vi "FILE READ FROM CSV.vi"(0 "File Path":string="C:\\data\\07_34_08_PM_01_July_2026\\07_34_08_PM_01_July_202607_34_08_PM_01_July_2026.csv", 5 "X-AXIS":u16(ring) items=["None", "Time ( Sec )", "Normal Load ( N )", "Frictional Force ( N )", "Coefficient of Friction", "Depth ( Microns )", "Speed ( RPM )", "Frequency ( Hz )", "Angle ( Degree )", "Cyclic Friction Force ( N )", "Cyclic Co efficient Friction ", "Stage temperature ( Degree celcius )", "Sample temperature ( Degree celcius )", "Stroke Length ( mm )", "Scratch Speed ( mm/sec )", "Amb Humidity ( % Rh ) ", "Amb Temperature (Deg C)", "Acoustic (mV)", "Mx (Nm)", "My (Nm)", "Mz (Nm)", "Humidity ( % Rh )", "Sliding Distance (mm)", "Wear Track Diameter (mm)", "Fx(N)", "Fy(N)", "MTM BallSpeed (RPM)", "MTM DiscSpeed (RPM)", "Entrainment Speed", "Slide Role", "Slip(%)", "Rotary Speed (m/sec)", "MTM Ball Speed (m/sec)", "MTM Disc Speed (m/sec)", "ECR (ohms)"], 9 "Y-AXIS":u16(ring) items=["None", "Time ( Sec )", "Normal Load ( N )", "Frictional Force ( N )", "Coefficient of Friction", "Depth ( Microns )", "Speed ( RPM )", "Frequency ( Hz )", "Angle ( Degree )", "Cyclic Friction Force ( N )", "Cyclic Co efficient Friction ", "Stage temperature ( Degree celcius )", "Sample temperature ( Degree celcius )", "Stroke Length ( mm )", "Scratch Speed ( mm/sec )", "Amb Humidity ( % Rh ) ", "Amb Temperature (Deg C)", "Acoustic (mV)", "Mx (Nm)", "My (Nm)", "Mz (Nm)", "Humidity ( % Rh )", "Sliding Distance (mm)", "Wear Track Diameter (mm)", "Fx(N)", "Fy(N)", "MTM BallSpeed (RPM)", "MTM DiscSpeed (RPM)", "Entrainment Speed", "Slide Role", "Slip(%)", "Rotary Speed (m/sec)", "MTM Ball Speed (m/sec)", "MTM Disc Speed (m/sec)", "ECR (ohms)"], 11 "error in (no error)":errorcluster) -> (4 "output cluster":cluster{"X":dbl[], "Y":dbl[]}, 6 "mean":dbl format="%0.2f", 8 "standard deviation":dbl format="%0.2f", 10 "variance":dbl format="%0.2f", 15 "error out":errorcluster)   [LabVIEW 2025]
uses:
  <vilib>/Analysis/NI_AALBase.lvlib
panel:
  # "C:\\data\\07_34_08_PM_01_July_2026\\07_34_08_PM_01_July_202607_34_08_PM_01_July_2026.csv"
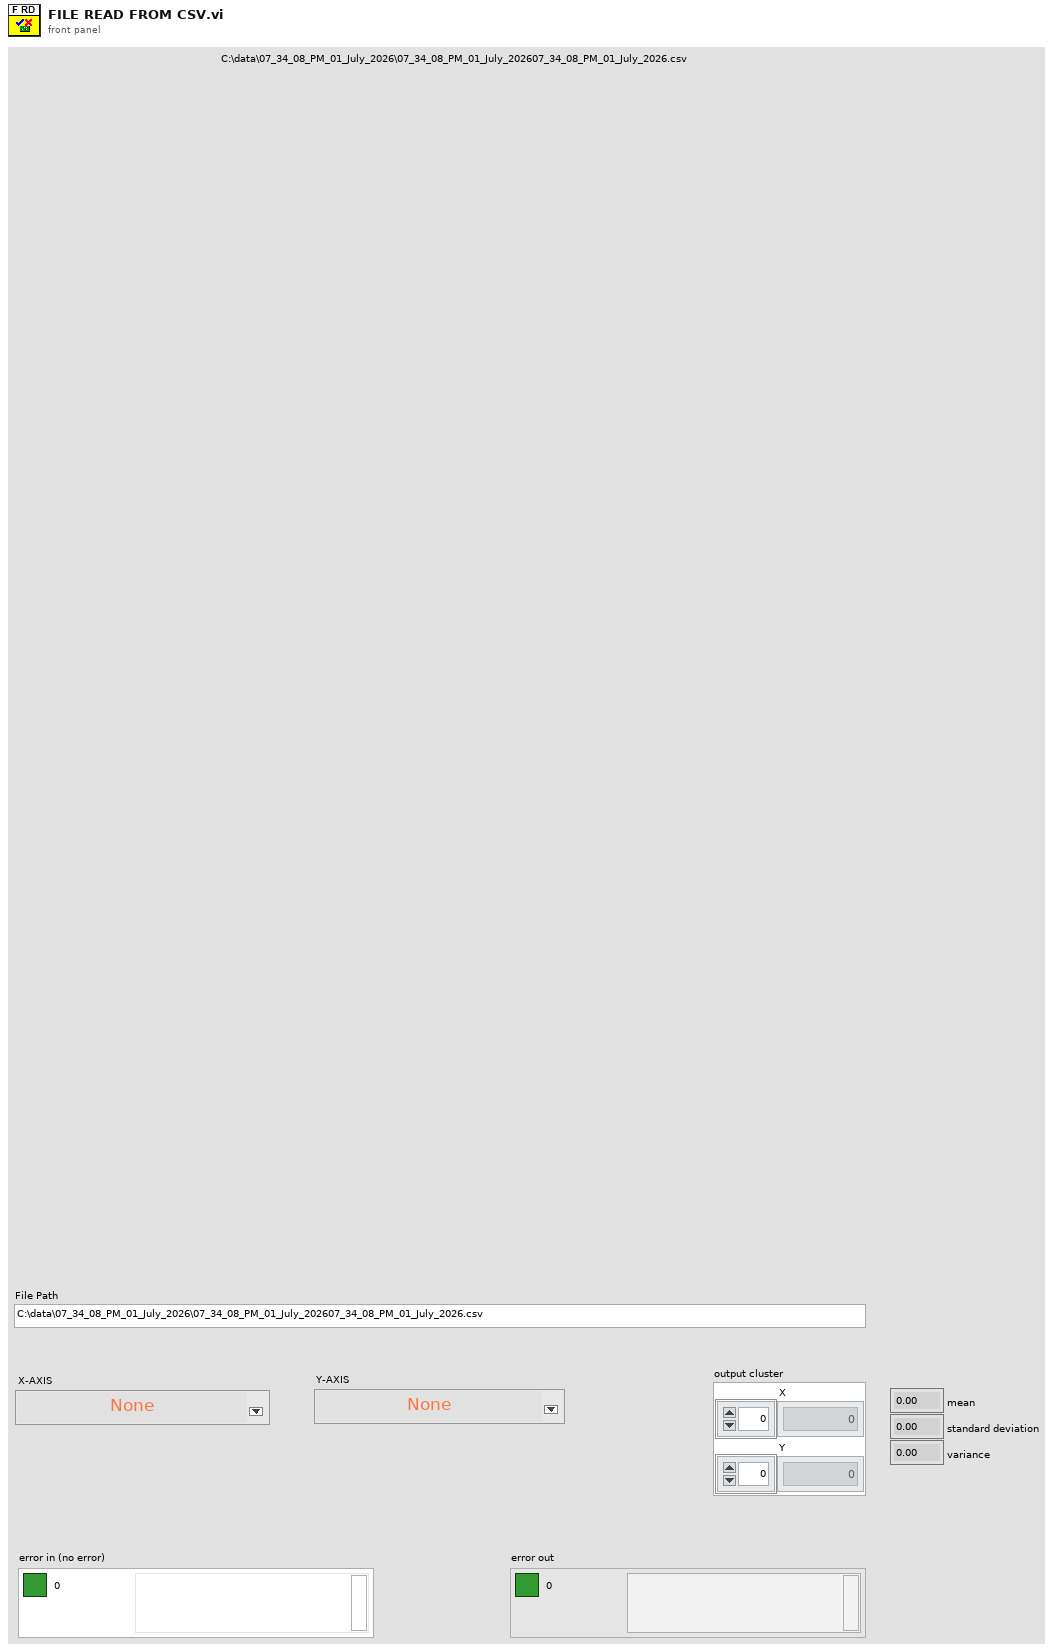
[diagram p1: front panel]
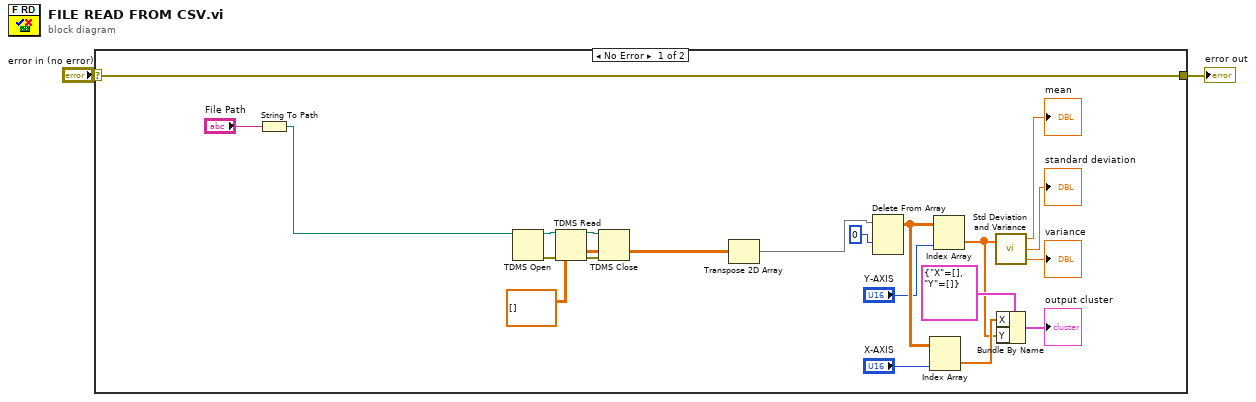
[diagram p0: block diagram]
diagram:
  n1 = case shown="No Error" "error in (no error)" {
    selector: "error in (no error)" -> [w15 _]
    tunnel: [w15 _] -> w1
    frame No Error {
      n2 = String To Path(string="File Path") -> (path=w3:path)
      n3 = TDMS Open(11:w3) -> (0:w10:errorcluster, 3:w9:refnum<k34>)  [unwired: 6 in]
      n4 = TDMS Read(0:w9, 11:w10, 12:dbl[][] []) -> (4:w7:refnum<k34>, 10:w5:dbl[][], 15:w8:errorcluster)  [unwired: 5 in, 3 out]
      n5 = TDMS Close(8:w8, 11:w7) -> ()  [unwired: 2 out]
      n6 = Transpose 2D Array(2D array=w5) -> (transposed array=w4:dbl[][])
      n7 = Delete From Array(array=w4, index (row)=0) -> (array with subset deleted=w20:dbl[][])  [unwired: 2 in, 1 out]
      n8 = Index Array(array=w20, index (col)="X-AXIS") -> (element=w17:dbl[])  [unwired: 1 in]
      n9 = Index Array(array=w20, index (col)="Y-AXIS") -> (element=w14:dbl[])  [unwired: 1 in]
      n10 = call <vilib>:"Std Deviation and Variance.vi"("X"=w14) -> ("mean"=→"mean":dbl, "standard deviation"=→"standard deviation":dbl, "variance"=→"variance":dbl)  [unwired: 1 in]
      n11 = Bundle By Name(cluster=cluster{"X":dbl[], "Y":dbl[]} {"X"=[], "Y"=[]} ("new element/subarray"), "X"=w17, "Y"=w14) -> (→"output cluster":cluster{"X":dbl[], "Y":dbl[]})
    }
    frame Error {
    }
  }
  "error out" <- w1
